vi "Close GUIs.vi"(0 "Windows":T1, 11 "error in (no error)":errorcluster) -> (15 "error out":errorcluster)   [LabVIEW 2019]
uses:
  TypeDef/Windows.ctl
  GUI Sensor Lib/GUI Sensor Lib.lvclass
  D:/GIT H4000/H4000/src/GUI_class/GUI.lvclass
  GUI Alarm Setting/GUI Alarm Setting.lvclass
  GUI Data Viewer_class/GUI Data Viewer.lvclass
  GUI Test Channels_class/GUI Test Channels.lvclass
  GUI Setting_class/GUI Setting.lvclass
  GUI Test HIPRESS_class/GUI Test HIPRESS.lvclass
  GUI NV class/GUI NV.lvclass
  GUI Work Windows_class/GUI Work Windows.lvclass
  PumpMotorGroup_class/GUI PumpMotorGroup.lvclass
  GUI_class/GUI.lvclass
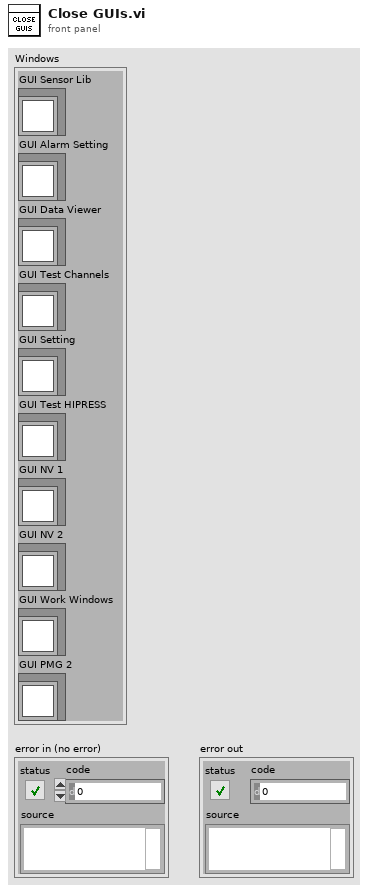
[diagram p1: front panel]
types:
  T1 = typedef "Windows.ctl" = cluster{"GUI Sensor Lib":refnum<class "GUI Sensor Lib.lvclass">, "GUI Alarm Setting":refnum<class "GUI Alarm Setting.lvclass">, "GUI Data Viewer":refnum<class "GUI Data Viewer.lvclass">, "GUI Test Channels":refnum<class "GUI Test Channels.lvclass">, "GUI Setting":refnum<class "GUI Setting.lvclass">, "GUI Test HIPRESS":refnum<class "GUI Test HIPRESS.lvclass">, "GUI NV 1":refnum<class "GUI NV.lvclass">, "GUI NV 2":refnum<class "GUI NV.lvclass">, "GUI Work Windows":refnum<class "GUI Work Windows.lvclass">, "GUI PMG 2":refnum<class "GUI PumpMotorGroup.lvclass">}
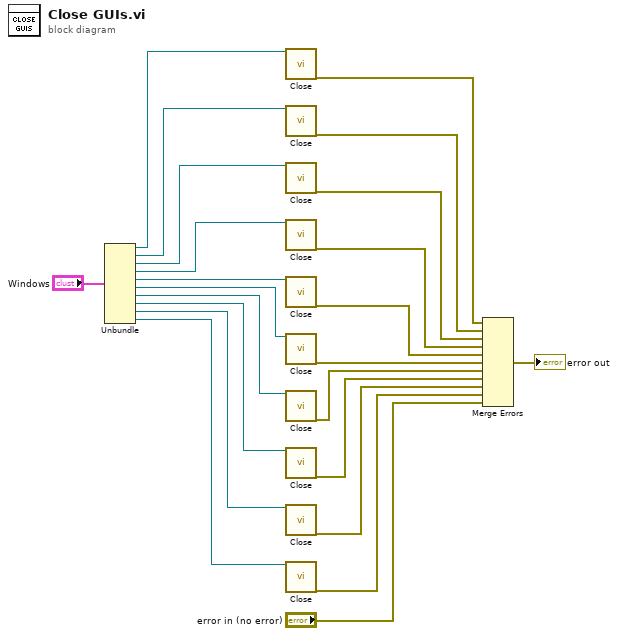
[diagram p0: block diagram]
diagram:
  n1 = Unbundle("Windows") -> ("GUI Sensor Lib"=w21:refnum<class "GUI Sensor Lib.lvclass">, "GUI Alarm Setting"=w19:refnum<class "GUI Alarm Setting.lvclass">, "GUI Data Viewer"=w17:refnum<class "GUI Data Viewer.lvclass">, "GUI Test Channels"=w15:refnum<class "GUI Test Channels.lvclass">, "GUI Setting"=w4:refnum<class "GUI Setting.lvclass">, "GUI Test HIPRESS"=w5:refnum<class "GUI Test HIPRESS.lvclass">, "GUI NV 1"=w6:refnum<class "GUI NV.lvclass">, "GUI NV 2"=w7:refnum<class "GUI NV.lvclass">, "GUI Work Windows"=w8:refnum<class "GUI Work Windows.lvclass">, "GUI PMG 2"=w14:refnum<class "GUI PumpMotorGroup.lvclass">)
  n2 = call "Close.vi"("reference in"=w21) -> ("error out"=w22:errorcluster)  [unwired: 16 in, 2 out]
  n3 = call "Close.vi"("reference in"=w19) -> ("error out"=w20:errorcluster)  [unwired: 16 in, 2 out]
  n4 = call "Close.vi"("reference in"=w17) -> ("error out"=w18:errorcluster)  [unwired: 16 in, 2 out]
  n5 = call "Close.vi"("reference in"=w15) -> ("error out"=w16:errorcluster)  [unwired: 16 in, 2 out]
  n6 = call "Close.vi"("reference in"=w4) -> ("error out"=w13:errorcluster)  [unwired: 16 in, 2 out]
  n7 = call "Close.vi"("reference in"=w5) -> ("error out"=w12:errorcluster)  [unwired: 16 in, 2 out]
  n8 = call "Close.vi"("reference in"=w6) -> ("error out"=w11:errorcluster)  [unwired: 16 in, 2 out]
  n9 = call "Close.vi"("reference in"=w7) -> ("error out"=w10:errorcluster)  [unwired: 16 in, 2 out]
  n10 = call "Close.vi"("reference in"=w8) -> ("error out"=w9:errorcluster)  [unwired: 16 in, 2 out]
  n11 = call "Close.vi"("reference in"=w14) -> ("error out"=w3:errorcluster)  [unwired: 16 in, 2 out]
  n12 = Merge Errors(w22, w20, w18, w16, w13, w12, w11, w10, w9, w3, "error in (no error)") -> (→"error out":errorcluster)
